vi "Set CSM LogtType Filter.vi"(10 "LogType":cluster{"CSM":string, "LogType":T1}[](array[cluster]), 11 "GlobalLogFilter in":refnum<class "GlobalLogFilter.lvclass">) -> (3 "GlobalLogFilter out":refnum<class "GlobalLogFilter.lvclass">)   [LabVIEW 2017, in "GlobalLogFilter.lvclass"]
uses:
  GlobalLogFilter.lvclass
  _Support/Typedef/_CSM_GlobalLog_MSG_TYPE.ctl
  GlobalLogFilter.lvclass/GlobalLogFilter.ctl
  Communicable State Machine.lvlib
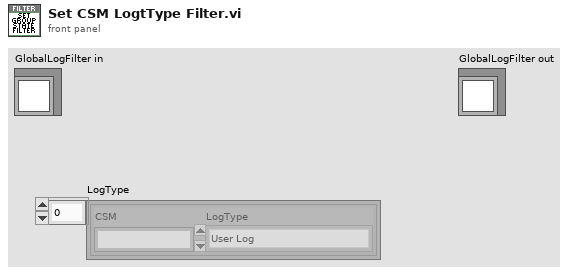
[diagram p1: front panel]
types:
  T1 = typedef "Communicable State Machine.lvlib/_CSM_GlobalLog_MSG_TYPE.ctl" = enum16{"User Log", "State Change", "Status", "Interrupt", "Register", "Unregister", "Error Log", "Module Created", "Module Destroyed"}
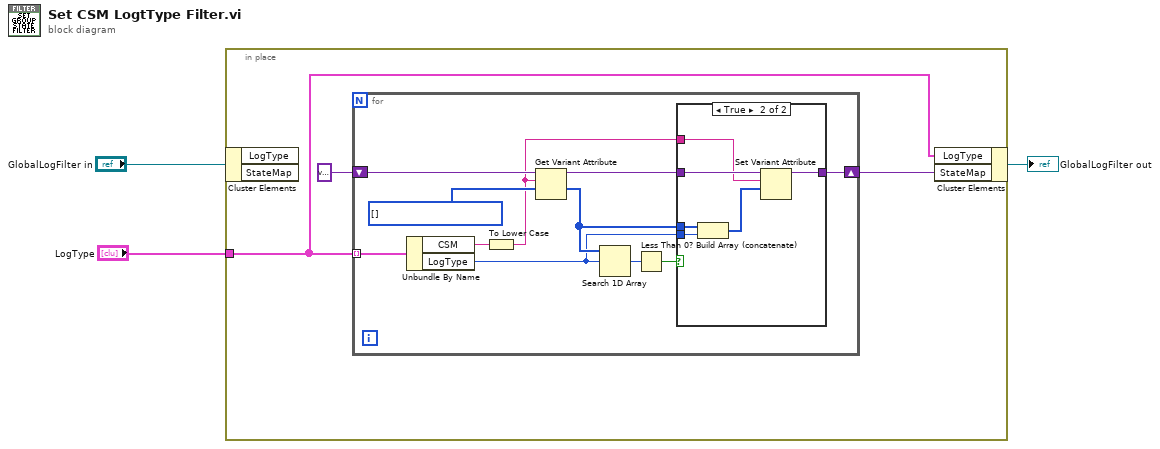
[diagram p0: block diagram]
diagram:
  n1 = in-place "In Place Element Structure" {
    in-place-border: "LogType" -> [w4]
    n2 = in-place-cluster #1("GlobalLogFilter in") -> ()  [unwired: 2 out]
    n3 = for {
      shift-right: [w10] -> w5
      shift-left: variant -> [w16]
      tunnel: w4 -> [w17] mode=indexing
      w14 = T1[] [] items=["User Log", "State Change", "Status", "Interrupt", "Register", "Unregister", "Error Log", "Module Created", "Module Destroyed"]
      n4 = Unbundle By Name(w17) -> ("CSM"=w9:string, "LogType"=w11:T1)
      n5 = To Lower Case(string=w9) -> (all lower case string=w7:string)
      n6 = Get Variant Attribute(Variant=w16, name=w7, default value (empty Variant)=w14) -> (duplicate Variant=w15:variant, value=w12:T1[])  [unwired: 1 in, 2 out]
      n7 = Search 1D Array(1D array=w12, element=w11) -> (index of element=w13:i32)  [unwired: 1 in]
      n8 = Less Than 0?(x=w13) -> (x < 0?=w8:bool)
      n9 = case shown="True" w8 {
        tunnel: w15 -> [w18 w24]
        tunnel: w12 -> [_ w23]
        tunnel: w11 -> [_ w22]
        tunnel: [w18 w21] -> w10
        tunnel: w7 -> [_ w19]
        frame False {
        }
        frame True {
          n10 = Build Array (concatenate)(w23, w22) -> (w20:T1[])
          n11 = Set Variant Attribute(Variant=w24, name=w19, value=w20) -> (Variant out=w21:variant)  [unwired: 1 in, 2 out]
        }
      }
    }
    n12 = in-place-cluster #1("LogType"=w4, "StateMap"=w5) -> (→"GlobalLogFilter out":refnum<class "GlobalLogFilter.lvclass">)
  }
